vi "AM_Rx_Template.vi"() -> ()   [LabVIEW 2013]
uses:
  <vilib>/Analysis/NI_AALBase.lvlib
  <instrlib>/niUSRP/niUSRP Fetch Rx Data (CDB WDT).vi
  <vilib>/Analysis/3filter.llb/Chebyshev Filter (CDB).vi
  <vilib>/Analysis/3filter.llb/Butterworth Filter (DBL).vi
panel:
  out "Rx AM Signal":waveform(dbl)(graph)
  out "Baseband Output":waveform(dbl)(graph)
  in  "stop":bool
  out "Error Out":errorcluster
  in  "Number of Samples":i64=200000
  in  "Active Antenna":string(combo)="RX2"
  out "Actual Gain (dB)":dbl format="%#_6f"
  in  "Gain (dB)":dbl format="%#_6f"
  out "Actual Frequency":dbl=100000.0 format="%#_6p"
  in  "Carrier Frequency":dbl=915000000.0 format="%#_6p"
  out "Actual IQ Rate":dbl=100000.0 format="%#_6p"
  in  "IQ Rate":dbl=1000000.0 format="%#_6p"
  in  "Device Names":refnum<k15>="192.168.10.2"
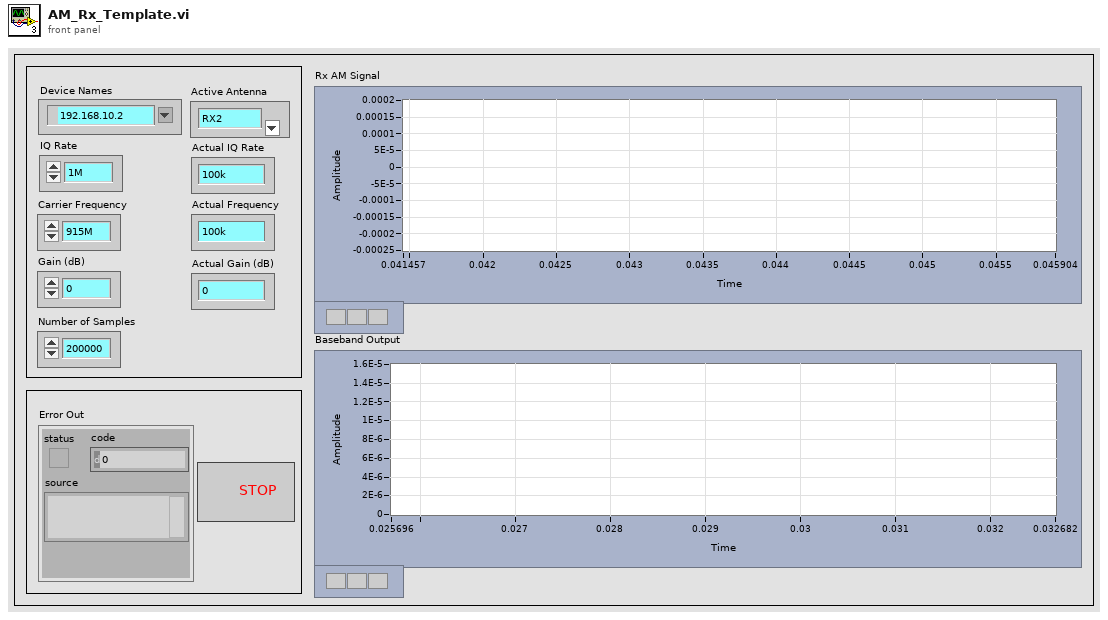
[diagram p1: front panel]
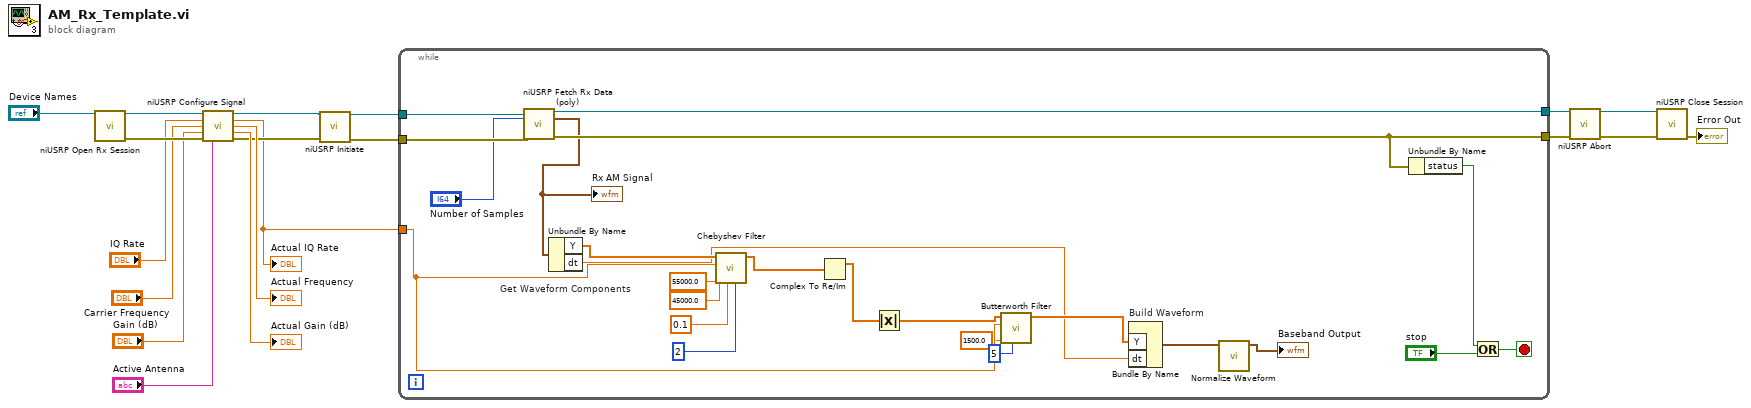
[diagram p0: block diagram]
diagram:
  n1 = call <instrlib>:"niUSRP Open Rx Session.vi"("device names"="Device Names") -> ("session handle out"=w18:refnum<k15>, "error out"=w17:errorcluster)  [unwired: 13 in]
  n2 = call <instrlib>:"niUSRP Configure Signal.vi"("session handle"=w18, "IQ rate"="IQ Rate", "carrier frequency"="Carrier Frequency", "gain"="Gain (dB)", "error in (no error)"=w17, "active antenna"="Active Antenna") -> ("session handle out"=w11:refnum<k15>, "coerced IQ rate"=w1:dbl, "coerced carrier frequency"=→"Actual Frequency":dbl, "coerced gain"=→"Actual Gain (dB)":dbl, "error out"=w10:errorcluster)  [unwired: 5 in]
  "Actual IQ Rate" <- w1
  n3 = call <instrlib>:"niUSRP Initiate.vi"("session handle"=w11, "error in (no error)"=w10) -> ("session handle out"=w8:refnum<k15>, "error out"=w7:errorcluster)  [unwired: 12 in]
  n4 = while {
    tunnel: w8 -> [w43]
    tunnel: w7 -> [w42]
    tunnel: [w41] -> w6
    tunnel: [w37] -> w5
    tunnel: w1 -> [w27]
    stop <- w40 stop-if-true
    n5 = call-poly <instrlib>:"niUSRP Fetch Rx Data (poly).vi"("session handle"=w43, "number of samples"="Number of Samples", "error in (no error)"=w42) -> ("session handle out"=w41:refnum<k15>, "data"=w23:waveform(cdb), "error out"=w37:errorcluster)  [unwired: 9 in, 1 out]
    "Rx AM Signal" <- w23
    n6 = Unbundle By Name "Get Waveform Components"(w23) -> ("Y"=w35:cdb[], "dt"=w20:dbl)
    n7 = call-poly <vilib>:"Chebyshev Filter.vi"("order"=2, "ripple(dB)"=0.1, "low cutoff freq: fl"=45000.0, "high cutoff freq: fh"=55000.0, "sampling freq: fs"=w27, "X"=w35) -> ("Filtered X"=w30:cdb[])  [unwired: 4 in, 1 out]
    n8 = Complex To Re/Im(x + iy=w30) -> (x=w29:dbl[])  [unwired: 1 out]
    n9 = Absolute Value(x=w29) -> (abs(x)=w28:dbl[])
    n10 = call-poly <vilib>:"Butterworth Filter.vi"("order"=5, "low cutoff freq: fl"=1500.0, "sampling freq: fs"=w27, "X"=w28) -> ("Filtered X"=w24:dbl[])  [unwired: 4 in, 1 out]
    n11 = Bundle By Name "Build Waveform"("Y"=w24, "dt"=w20) -> (w22:waveform(dbl))  [unwired: 1 in]
    n12 = call <vilib>:"Normalize Waveform.vi"("waveform in"=w22) -> ("normalized waveform"=→"Baseband Output":waveform(dbl))  [unwired: 7 in, 3 out]
    n13 = Unbundle By Name(w37) -> ("status"=w39:bool)
    n14 = Or(x=w39, y="stop") -> (x .or. y?=w40:bool)
  }
  n15 = call <instrlib>:"niUSRP Abort.vi"("session handle"=w6, "error in (no error)"=w5) -> ("session handle out"=w4:refnum<k15>, "error out"=w3:errorcluster)  [unwired: 12 in]
  n16 = call <instrlib>:"niUSRP Close Session.vi"("session handle"=w4, "error in (no error)"=w3) -> ("error out"=→"Error Out":errorcluster)  [unwired: 13 in]
